vi "Create Server.vi"(5 "Server Key File (.key)":path, 7 "Server Certificate File (.crt)":path, 8 "error in":errorcluster, 11 "Server Address":string) -> (0 "error out":errorcluster, 3 "gRPC Server out":refnum<class "Servicer.lvclass">)   [LabVIEW 2019, in "gRPC-servicer.lvlib" / "Servicer.lvclass"]
uses:
  Servicer.lvclass
  Servicer.lvclass/Servicer.ctl
  gRPC lv Support/grpc-lvsupport/grpc-lvsupport.lvlib
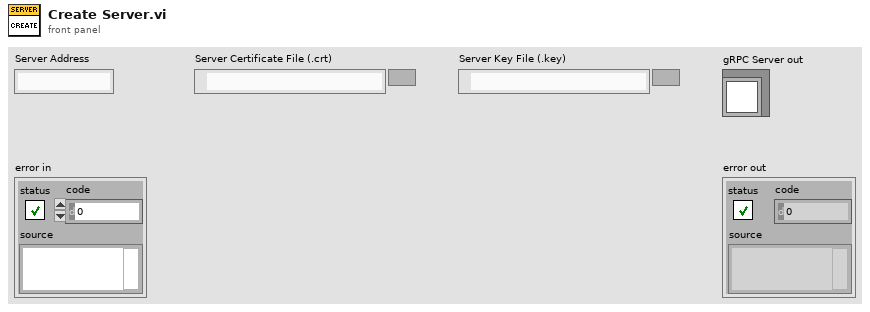
[diagram p1: front panel]
types:
  T1 = typedef "grpc-lvsupport.lvlib/grpcId.ctl" = u64
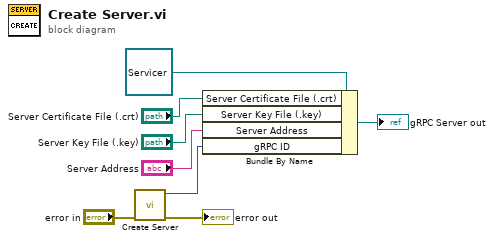
[diagram p0: block diagram]
diagram:
  n1 = call "Create Server.vi"("error in"="error in") -> ("error out"=→"error out":errorcluster, "gRPCid out"=w3:T1)  [unwired: 9 in]
  n2 = Bundle By Name(cluster=refnum<class "Servicer.lvclass"> refnum ("OOP Server out"), "Server Certificate File (.crt)"="Server Certificate File (.crt)", "Server Key File (.key)"="Server Key File (.key)", "Server Address"="Server Address", "gRPC ID"=w3) -> (→"gRPC Server out":refnum<class "Servicer.lvclass">)
